vi "MSFET208_Input&Output.vi"(0 "Data Saved in":path=path "C:/Users/Garrett/Google Drive/Documents/Martz Lab/LabView/pH_Sensor project/pH_Voltages208.csv", 1 "Sensor in":string(combo)="MSFET 208", 3 "Boolean":bool, 4 "Weighting (Sample)":enum16{"Sample", "Population"}(ring), 5 "Temp Voltage":dbl[](array[numeric]) format="%0.2f", 6 "ISFET Voltage":dbl[](array[numeric]), 7 "REF voltage":dbl[](array[numeric]), 9 "DirecTemp":dbl=23.4) -> (12 "MS 208 Temp":dbl=24.4655047055293, 13 "Mean3":dbl=nan format="%.5f", 14 "std2":dbl=nan format="%.5f", 15 "Mean2":dbl=nan format="%.5f", 18 "std3":dbl=nan format="%.5f", 19 "pHint":dbl=39.163636363636364)   [LabVIEW 2018]
uses:
  <vilib>/Utility/file.llb/Write Delimited Spreadsheet (string).vi
  <vilib>/Analysis/NI_AALBase.lvlib
panel:
  out "std1 2":dbl=0.00039728728704078564 format="%.5f"
  out "Mean1 2":dbl=1.408027196389114 format="%.5f"
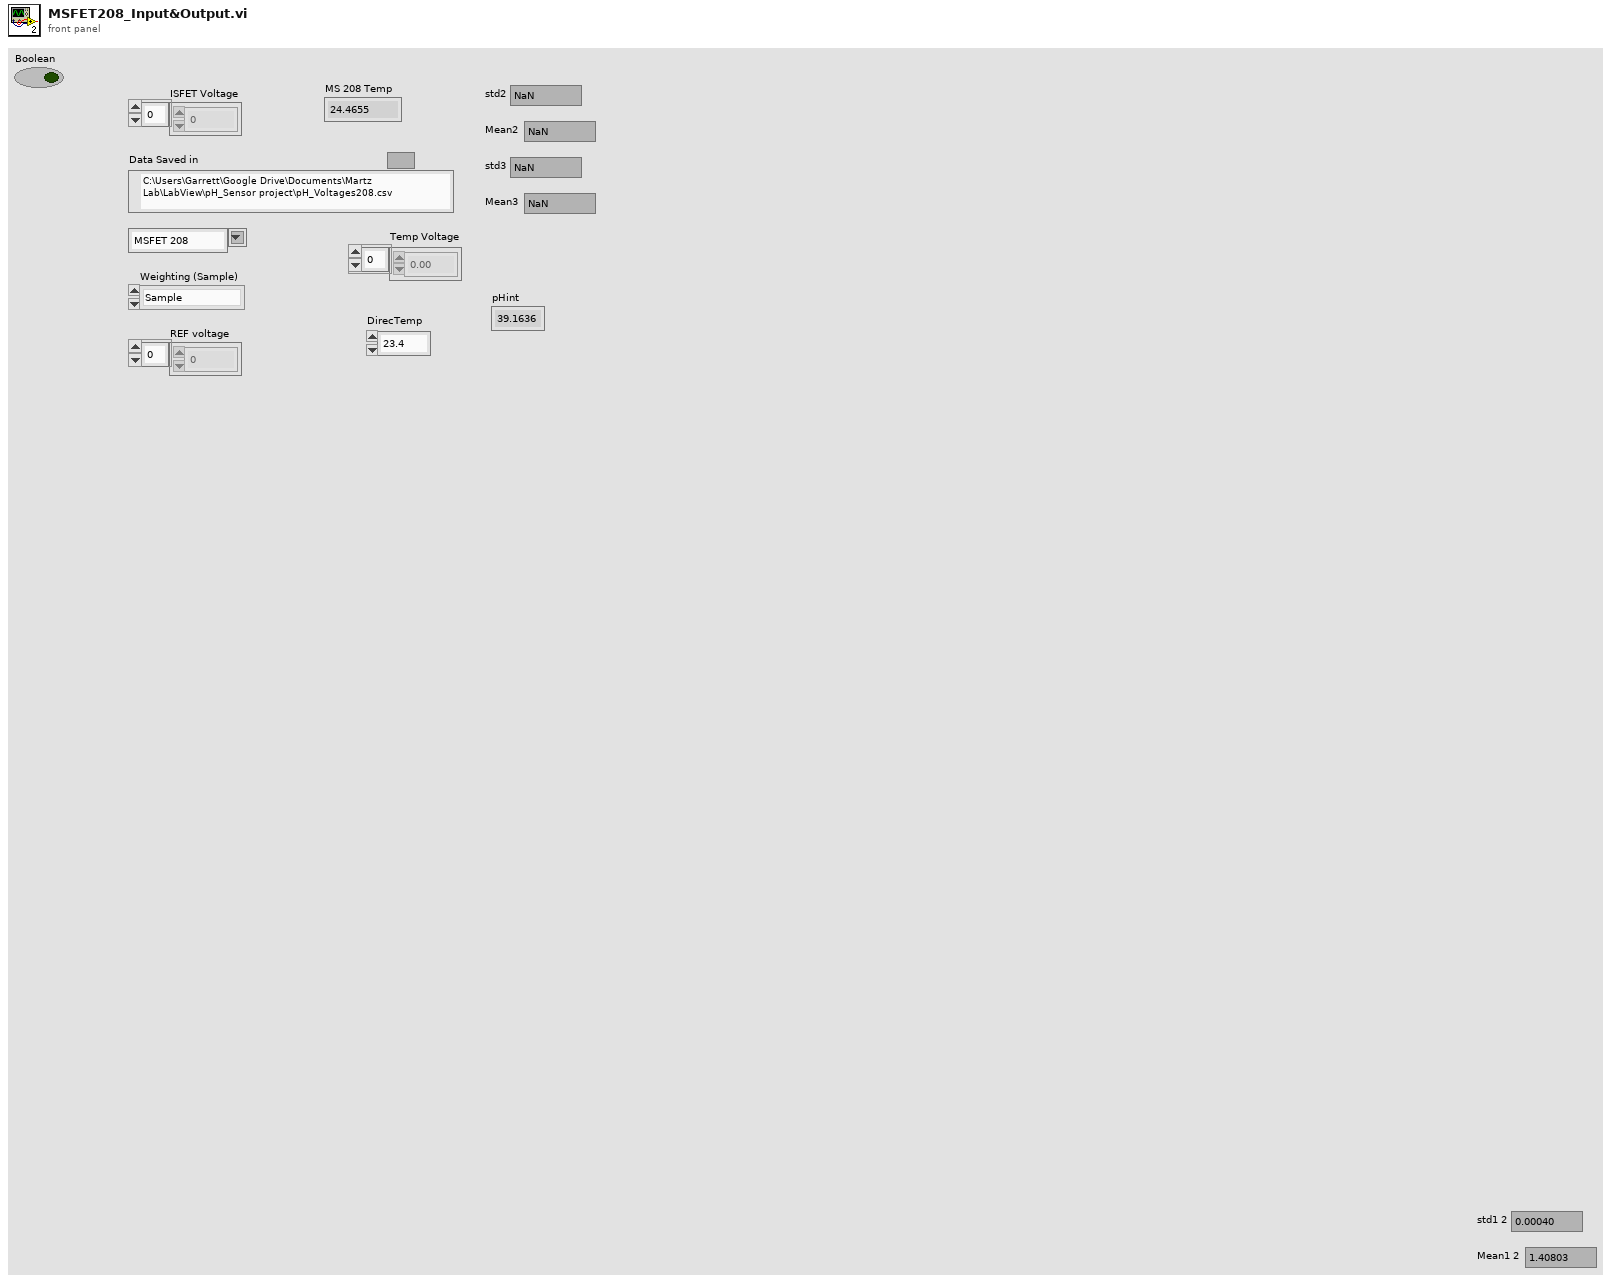
[diagram p1: front panel]
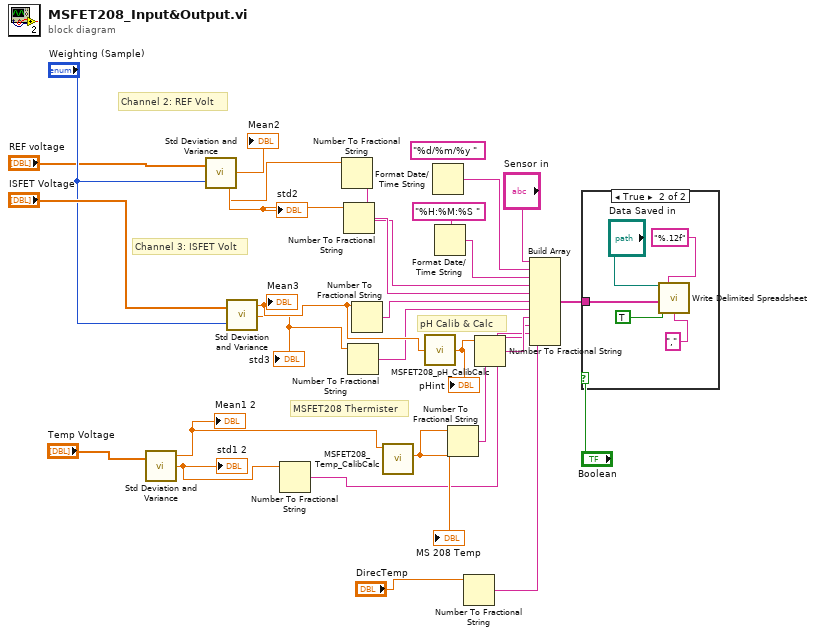
[diagram p0: block diagram]
diagram:
  (unwired) "%d/%m/%y " ("time format string (%c)")
  # "MSFET208 Thermister"
  # "pH Calib & Calc"
  # "Channel 3: ISFET Volt"
  # "Channel 2: REF Volt"
  n1 = call <vilib>:"Std Deviation and Variance.vi"("X"="Temp Voltage") -> ("mean"=w8:dbl, "standard deviation"=w9:dbl)  [unwired: 1 in, 1 out]
  "Mean1 2" <- w8
  "std1 2" <- w9
  n2 = call <vilib>:"Std Deviation and Variance.vi"("X"="REF voltage", "Weighting (Sample)"="Weighting (Sample)") -> ("mean"=w14:dbl, "standard deviation"=w17:dbl)  [unwired: 1 out]
  "Mean2" <- w14
  "std2" <- w17
  n3 = call <vilib>:"Std Deviation and Variance.vi"("X"="ISFET Voltage", "Weighting (Sample)"="Weighting (Sample)") -> ("mean"=w24:dbl, "standard deviation"=w20:dbl)  [unwired: 1 out]
  "Mean3" <- w24
  "std3" <- w20
  n4 = Number To Fractional String(number=w9) -> (F-format string=w4:string)  [unwired: 3 in]
  n5 = Number To Fractional String(number=w14) -> (F-format string=w16:string)  [unwired: 3 in]
  n6 = Number To Fractional String(number=w17) -> (F-format string=w18:string)  [unwired: 3 in]
  n7 = Number To Fractional String(number=w20) -> (F-format string=w21:string)  [unwired: 3 in]
  n8 = Number To Fractional String(number=w24) -> (F-format string=w19:string)  [unwired: 3 in]
  n9 = call "MSFET208_Temp_CalibCalc.vi"("Voltage from Thermistor"=w8) -> ("Temperature (C)"=w7:dbl)  [unwired: 10 in]
  "MS 208 Temp" <- w7
  n10 = call "MSFET208_pH_CalibCalc.vi"("Eint"=w24) -> ("pHint"=w22:dbl)
  "pHint" <- w22
  n11 = Format Date/Time String() -> (date/time string=w26:string)  [unwired: 3 in]
  n12 = Format Date/Time String(time format string (%c)="%H:%M:%S ") -> (date/time string=w27:string)  [unwired: 2 in]
  n13 = Number To Fractional String(number=w7) -> (F-format string=w5:string)  [unwired: 3 in]
  n14 = Number To Fractional String(number="DirecTemp") -> (F-format string=w1:string)  [unwired: 3 in]
  n15 = Number To Fractional String(number=w22) -> (F-format string=w23:string)  [unwired: 3 in]
  n16 = Build Array("Sensor in", w26, w27, w16, w18, w19, w21, w23, w5, w4, w1) -> (w13:string[])
  n17 = case shown="True" "Boolean" {
    tunnel: w13 -> [_ w28]
    frame False {
    }
    frame True {
      n18 = call-poly <vilib>:"Write Delimited Spreadsheet.vi"("file path (dialog if empty)"="Data Saved in", "format (%s)"="%.12f" ("format (%.3f)"), "1D data"=w28, "append to file? (new file:F)"=TRUE, "delimiter (\\t)"="," ("delimiter (\\t)")) -> ()  [unwired: 9 in, 2 out]
    }
  }
